vi "CRYUnflatten Data SC.vi"(10 "Unflatten data":string) -> (0 "Error?":bool, 2 "Data out":T3={"Name"="", "Curve"=[], "X data"=1, "Y data"=1, "Z data"=1, "X axis"=0, "Y axis"=1, "Z axis"=1, "X unit"="Hz", "Y unit"="", "Z unit"="deg.", "X dB ref"=1.0, "Y dB ref"=1.0, "Z dB ref"=1.0, "single val"=FALSE, "protected"=FALSE, "display X"=TRUE, "display Y"=TRUE, "display Z"=TRUE, "Plot Settings"={"Color"=0, "Interpolation"=2, "Point Style"=0, "Line Style"=0, "Point Color"=0, "Line Width"=0, "Bar Plot Style"=0, "Fill To"=-1}, "Test Info"=""} {"Z data" items=["dB", "Lin", "Pwr"]; "X data" items=["dB", "Lin", "Pwr"]; "Y data" items=["dB", "Lin", "Pwr"]; "Z dB ref" format="%.1f"; "Z axis" items=["Log", "Lin"]; "X dB ref" format="%.1f"; "X axis" items=["Log", "Lin"]; "Y axis" items=["Log", "Lin"]; "Y dB ref" format="%.1f"; "Curve"."z" format="%.2f"; "Curve"."y" format="%.2f"; "Curve"."x" format="%.2f"}, 3 "Header info out":T5={"Data type"="Data            ", "Version"=1, "Dimensions"=0, "Curve name"="Data            ", "Reserved"="Data            "})   [LabVIEW 2013]
uses:
  Typedef Control/CRYData Cluster SC.ctl
  Typedef Control/CRYAxis Unit Type.ctl
panel:
  in  "Datum 2.0":T1={"curve name"="", "Curve"=[], "Xdata"=0, "Ydata"=0, "Zdata"=0, "Xaxis"=0, "Yaxis"=0, "Zaxis"=0, "Xunit Prefix"="", "Yunit Prefix"="", "Zunit Prefix"="", "Xunit name"="", "Yunit name"="", "Zunit name"="", "X dB ref"=1.0, "Y dB ref"=1.0, "Z dB ref"=1.0, "single val"=FALSE} {"Z dB ref" format="%.1f"; "Y dB ref" format="%.1f"; "X dB ref" format="%.1f"; "Curve"."z" format="%.2f"; "Curve"."y" format="%.2f"; "Curve"."x" format="%.2f"}
  in  "Datum 3.0":T2={"curve name"="", "Curve"=[], "Xdata"=0, "Ydata"=0, "Zdata"=0, "Xaxis"=0, "Yaxis"=0, "Zaxis"=0, "Xunit Prefix"="", "Yunit Prefix"="", "Zunit Prefix"="", "Xunit name"="", "Yunit name"="", "Zunit name"="", "X dB ref"=1.0, "Y dB ref"=1.0, "Z dB ref"=1.0, "single val"=FALSE, "protected"=FALSE, "display X"=TRUE, "display Y"=TRUE, "display Z"=TRUE, "Plot Settings"={"Color"=0}} {"Z dB ref" format="%.1f"; "Y dB ref" format="%.1f"; "X dB ref" format="%.1f"; "Curve"."z" format="%.2f"; "Curve"."y" format="%.2f"; "Curve"."x" format="%.2f"}
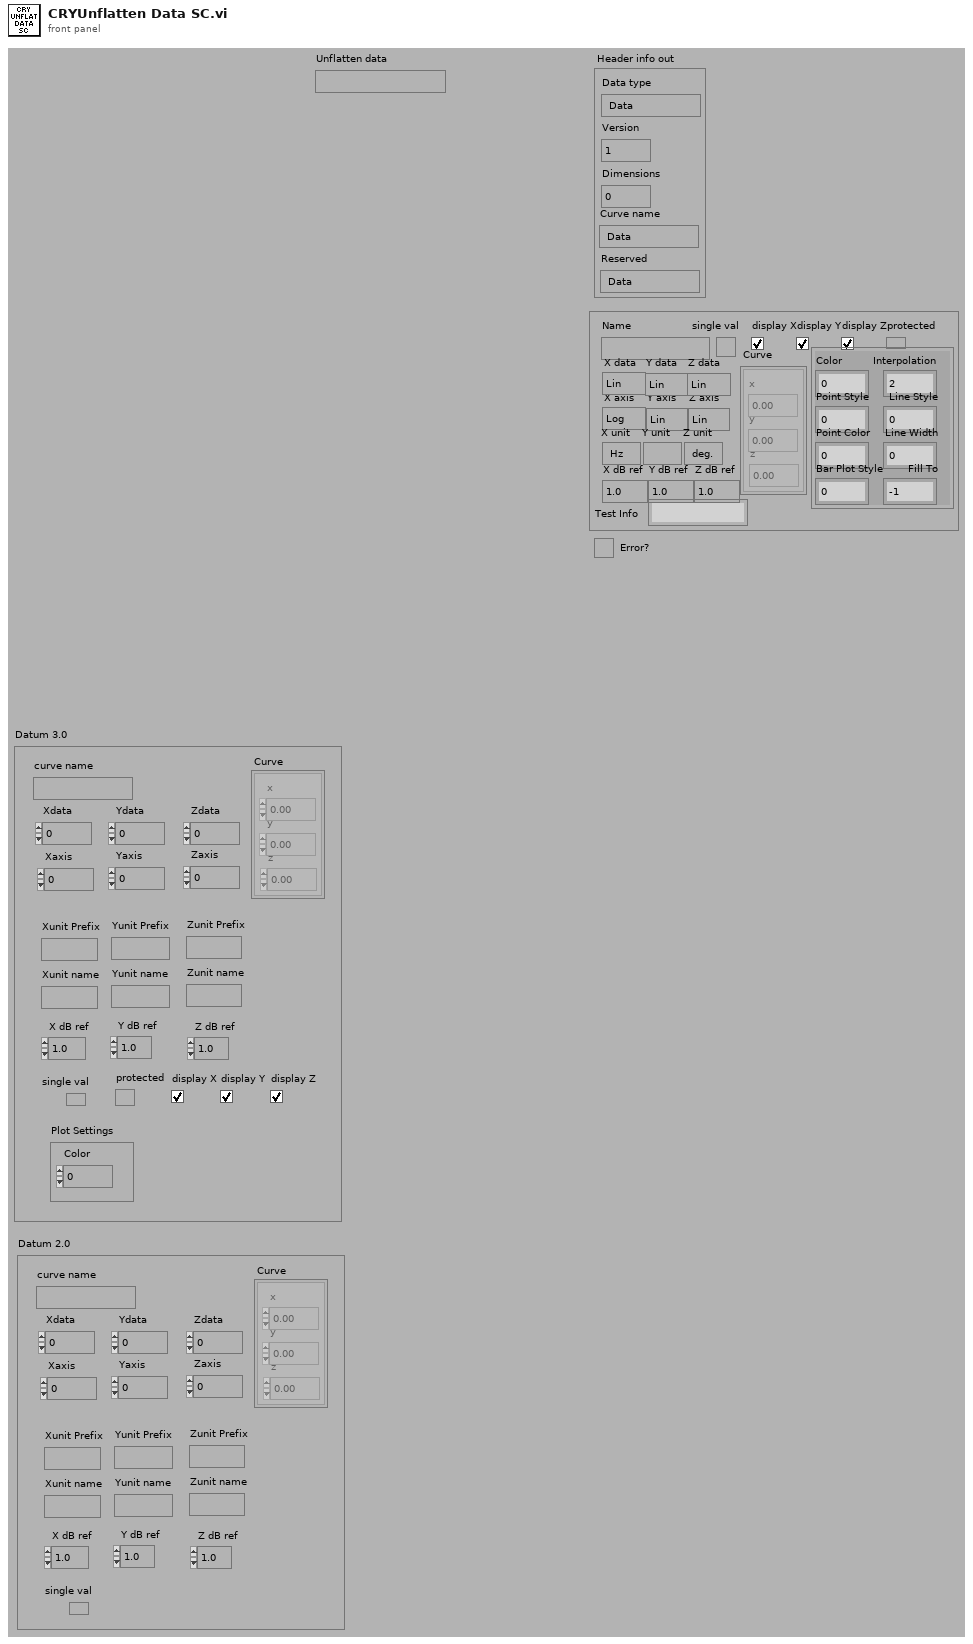
[diagram p1: front panel]
types:
  T1 = cluster{"curve name":string, "Curve":cluster{"x":dbl, "y":dbl, "z":dbl}[], "Xdata":u16, "Ydata":u16, "Zdata":u16, "Xaxis":u16, "Yaxis":u16, "Zaxis":u16, "Xunit Prefix":string, "Yunit Prefix":string, "Zunit Prefix":string, "Xunit name":string, "Yunit name":string, "Zunit name":string, "X dB ref":dbl, "Y dB ref":dbl, "Z dB ref":dbl, "single val":bool}
  T2 = cluster{"curve name":string, "Curve":cluster{"x":dbl, "y":dbl, "z":dbl}[], "Xdata":u16, "Ydata":u16, "Zdata":u16, "Xaxis":u16, "Yaxis":u16, "Zaxis":u16, "Xunit Prefix":string, "Yunit Prefix":string, "Zunit Prefix":string, "Xunit name":string, "Yunit name":string, "Zunit name":string, "X dB ref":dbl, "Y dB ref":dbl, "Z dB ref":dbl, "single val":bool, "protected":bool, "display X":bool, "display Y":bool, "display Z":bool, "Plot Settings":cluster{"Color":u32}}
  T3 = typedef "CRYData Cluster SC.ctl" = cluster{"Name":string, "Curve":cluster{"x":dbl, "y":dbl, "z":dbl}[], "X data":T4, "Y data":T4, "Z data":T4, "X axis":u16, "Y axis":u16, "Z axis":u16, "X unit":string, "Y unit":string, "Z unit":string, "X dB ref":dbl, "Y dB ref":dbl, "Z dB ref":dbl, "single val":bool, "protected":bool, "display X":bool, "display Y":bool, "display Z":bool, "Plot Settings":cluster{"Color":u32, "Interpolation":u8, "Point Style":u8, "Line Style":u8, "Point Color":u32, "Line Width":u8, "Bar Plot Style":u8, "Fill To":i16}, "Test Info":string}
  T4 = typedef "CRYAxis Unit Type.ctl" = u16
  T5 = cluster{"Data type":string, "Version":u16, "Dimensions":u8, "Curve name":string, "Reserved":string}
  T6 = cluster{"curve name":string, "Curve":cluster{"x":dbl, "y":dbl, "z":dbl}[], "Xdata":u16, "Ydata":u16, "Zdata":u16, "Xaxis":u16, "Yaxis":u16, "Zaxis":u16, "Xunit name":string, "Yunit name":string, "Zunit name":string, "X dB ref":dbl, "Y dB ref":dbl, "Z dB ref":dbl, "single val":bool, "protected":bool, "display X":bool, "display Y":bool, "display Z":bool, "Plot Settings":cluster{"Color":u32, "Interpolation":u8, "Point Style":u8, "Line Style":u8, "Point Color":u32, "Line Width":u8, "Bar Plot Style":u8, "Fill To":i16}, "Test Info":string}
  T7 = cluster{"Color":u32, "Interpolation":u8, "Point Style":u8, "Line Style":u8, "Point Color":u32, "Line Width":u8, "Bar Plot Style":u8, "Fill To":i16}
  T8 = cluster{"unsigned byte array[0]":u8, "unsigned byte array[1]":u8, "unsigned byte array[2]":u8}
  T9 = cluster{"substring":string, u16, "unsigned byte array[2]":u8, "Unflatten data":string, "Unflatten data":string}
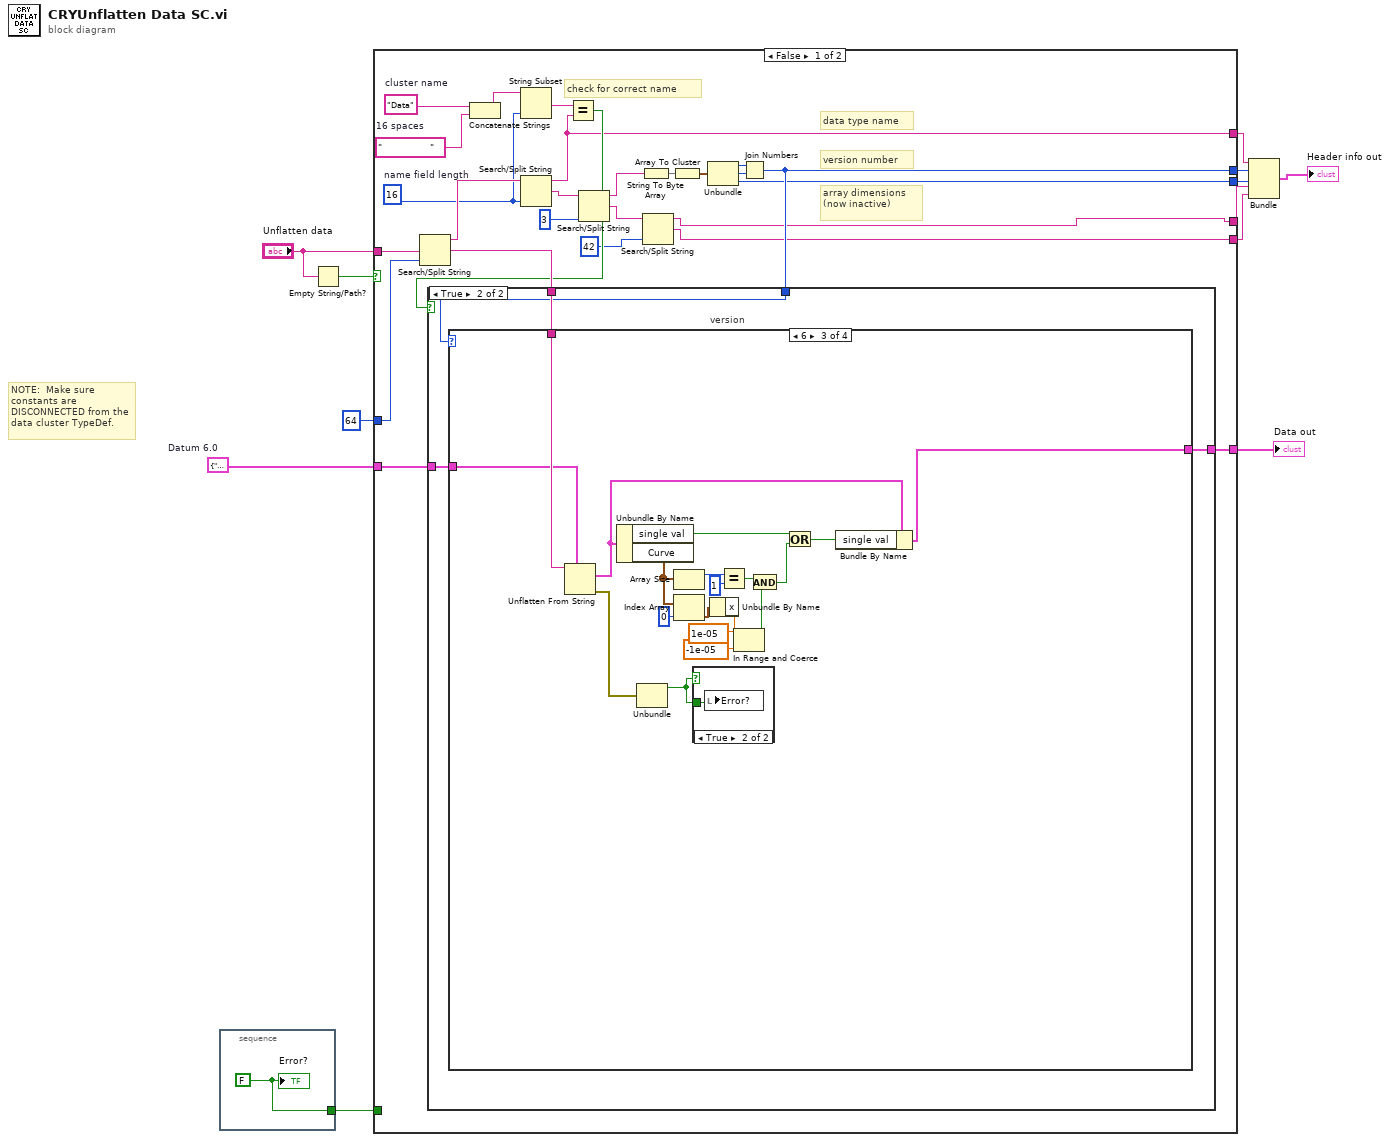
[diagram p0: block diagram]
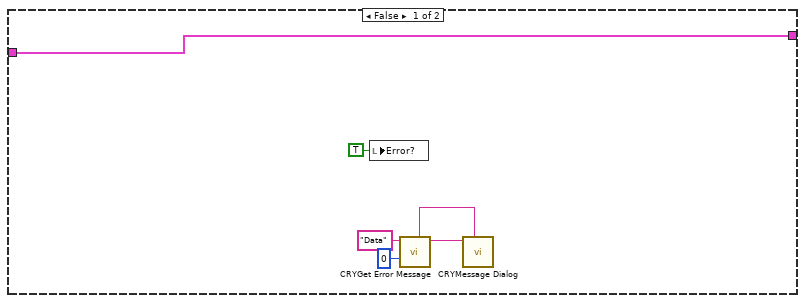
[diagram p2: hidden frame]
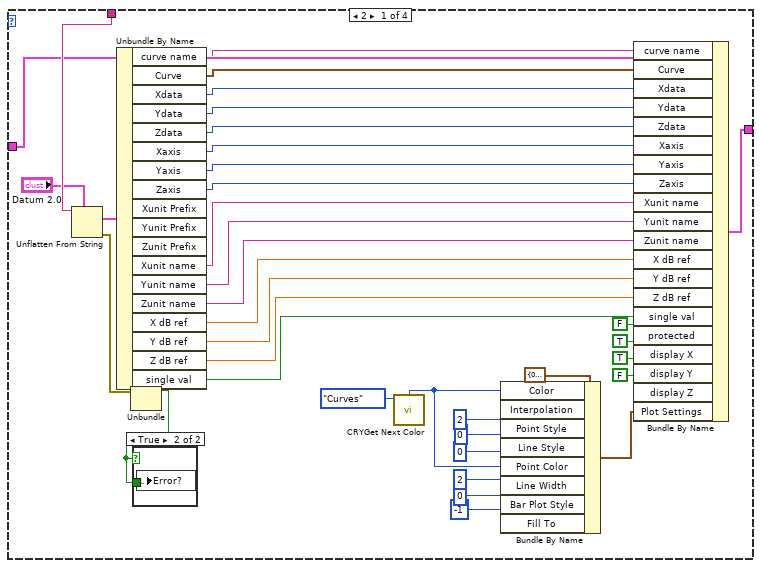
[diagram p3: hidden frame]
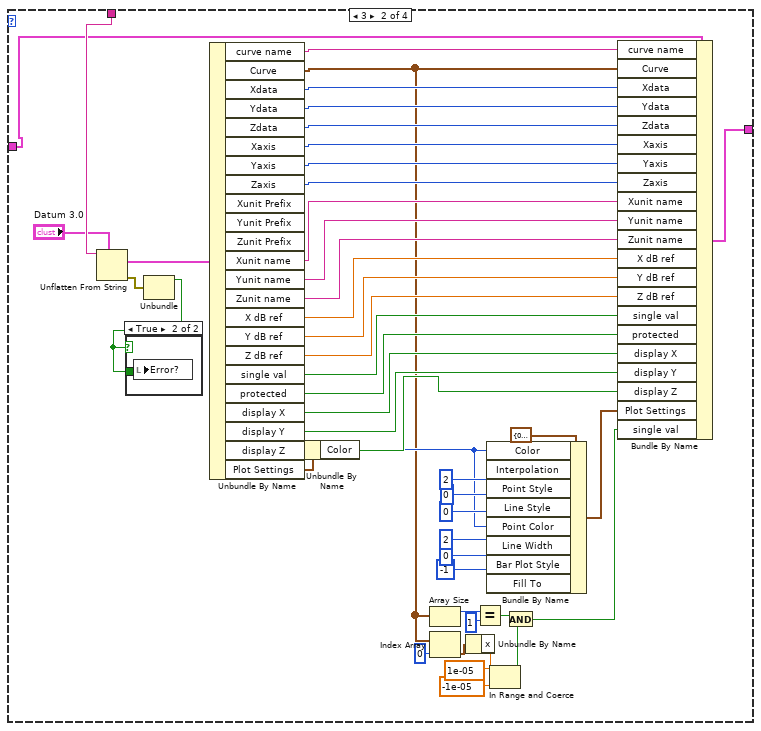
[diagram p5: hidden frame]
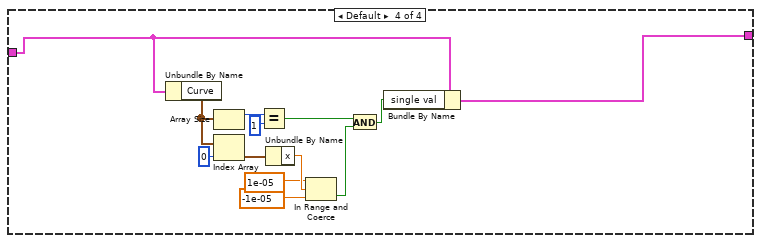
[diagram p8: hidden frame]
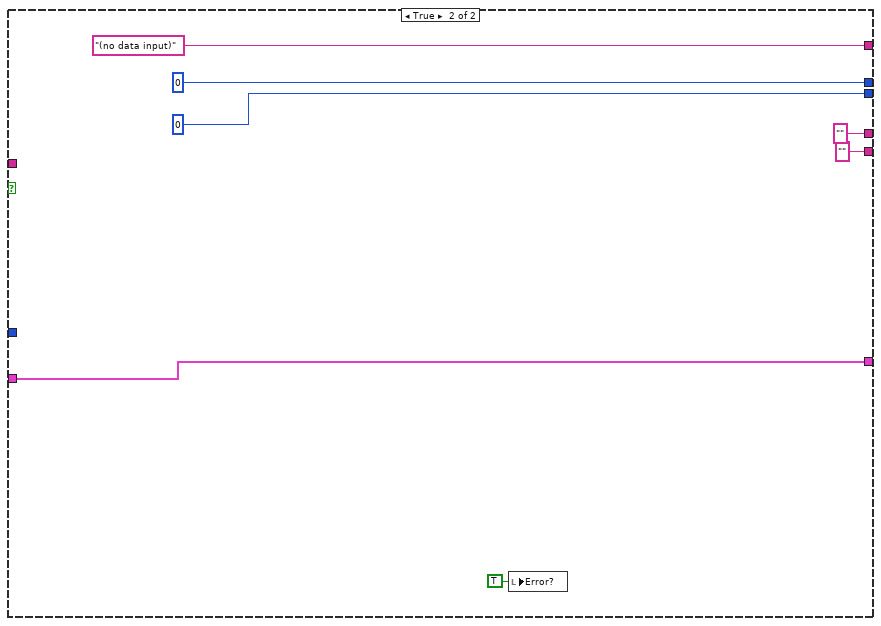
[diagram p9: hidden frame]
diagram:
  w2 = T6 {"curve name"="", "Curve"=[], "Xdata"=0, "Ydata"=0, "Zdata"=0, "Xaxis"=0, "Yaxis"=0, "Zaxis"=0, "Xunit name"="", "Yunit name"="", "Zunit name"="", "X dB ref"=0.0, "Y dB ref"=0.0, "Z dB ref"=0.0, "single val"=FALSE, "protected"=FALSE, "display X"=FALSE, "display Y"=FALSE, "display Z"=FALSE, "Plot Settings"={"Color"=0, "Interpolation"=0, "Point Style"=0, "Line Style"=0, "Point Color"=0, "Line Width"=0, "Bar Plot Style"=0, "Fill To"=0}, "Test Info"=""}  # Datum 6.0
  # "NOTE:  Make sure constants are DISCONNECTED from the data cluster TypeDef."
  n1 = stacked-sequence {
    tunnel: [w13] -> w1
    frame #0 {
      w13 = FALSE
      "Error?" <- w13
    }
  }
  n2 = Empty String/Path?(string/path="Unflatten data") -> (empty?=w11:bool)
  n3 = case shown="False" w11 {
    tunnel: "Unflatten data" -> [w39 _]
    tunnel: 64 ("header length") -> [w33 _]
    tunnel: [w30 u16 0] -> w8
    tunnel: [w23 u8 0] -> w9
    tunnel: [w24 "(no data input)" ("substring")] -> w7
    tunnel: [w22 w170] -> w3
    tunnel: w2 -> [w21 w170]
    tunnel: [w15 "" ("Unflatten data")] -> w5
    tunnel: [w14 "" ("Unflatten data")] -> w4
    tunnel: w1 -> [_ _]
    frame False {
      w28 = "                "  # 16 spaces
      w29 = "Data"  # cluster name
      w26 = 16  # name field length
      # "check for correct name"
      # "array dimensions\n(now inactive)"
      # "version number"
      # "data type name"
      n4 = Search/Split String(string=w39, offset (0)=w33) -> (substring before match=w32:string, match + rest of string=w34:string)  [unwired: 2 out]
      n5 = Concatenate Strings(w29, w28) -> (w27:string)
      n6 = String Subset(string=w27, length (rest)=w26) -> (substring=w25:string)  [unwired: 1 out]
      n7 = Search/Split String(string=w32, offset (0)=w26) -> (substring before match=w24:string, match + rest of string=w20:string)  [unwired: 2 out]
      n8 = Equal?(x=w25, y=w24) -> (x = y?=w31:bool)
      n9 = Search/Split String(string=w20, offset (0)=3 ("name field length")) -> (substring before match=w18:string, match + rest of string=w17:string)  [unwired: 2 out]
      n10 = String To Byte Array(string=w18) -> (unsigned byte array=w38:u8[])
      n11 = Search/Split String(string=w17, offset (0)=42 ("name field length")) -> (substring before match=w15:string, match + rest of string=w14:string)  [unwired: 2 out]
      n12 = Array To Cluster(array=w38) -> (cluster=w37:T8)
      n13 = Unbundle(w37) -> ("unsigned byte array[0]"=w36:u8, "unsigned byte array[1]"=w35:u8, "unsigned byte array[2]"=w23:u8)
      n14 = Join Numbers(hi=w36, lo=w35) -> ((hi.lo)=w30:u16)
      n15 = case shown="True" w31 {
        tunnel: w34 -> [_ w49]
        tunnel: w30 -> [_ w48]
        tunnel: [w45 w47] -> w22
        tunnel: w21 -> [w45 w46]
        frame False {
          n16 = local write "Error?"(TRUE ("Error?")) -> ()
          n17 = call "CRYGet Error Message.vi"("Error No"=0, "Kind"="Data") -> ("Message"=w43:string, "Window Title"=w44:string)  [unwired: 4 in, 4 out]
          n18 = call "CRYMessage Dialog.vi"("Window Title"=w44, "Message Content"=w43) -> ()  [unwired: 8 in, 2 out]
        }
        frame True {
          n19 = case "version" shown="6" w48 {
            tunnel: w49 -> [w85 w132 w137 _]
            tunnel: [w68 w110 w136 w154] -> w47
            tunnel: w46 -> [w83 w129 w135 w155]
            frame 2 {
              n20 = Unflatten From String(type="Datum 2.0", binary string=w85) -> (value=w84:T1, error out=w50:errorcluster)  [unwired: 1 in, 3 out]
              n21 = Unbundle By Name(w84) -> ("curve name"=w82:string, "Curve"=w81:cluster{"x":dbl, "y":dbl, "z":dbl}[], "Xdata"=w80:u16, "Ydata"=w79:u16, "Zdata"=w78:u16, "Xaxis"=w77:u16, "Yaxis"=w76:u16, "Zaxis"=w75:u16, "Xunit name"=w74:string, "Yunit name"=w73:string, "Zunit name"=w72:string, "X dB ref"=w71:dbl, "Y dB ref"=w70:dbl, "Z dB ref"=w62:dbl, "single val"=w69:bool)  [unwired: 3 out]
              n22 = Unbundle(w50) -> ("status"=w51:bool)  [unwired: 2 out]
              n23 = case shown="True" w51 {
                tunnel: w51 -> [_ w86]
                frame False {
                }
                frame True {
                  n24 = local write "Error?"(w86) -> ()
                }
              }
              n25 = call "CRYGet Next Color.vi"("Type"=enum16{"Curves", "Values", "Results", "WFM"}."Curves") -> ("Color"=w53:u32)  [unwired: 10 out]
              n26 = Bundle By Name(cluster=T7 {"Color"=0, "Interpolation"=0, "Point Style"=0, "Line Style"=0, "Point Color"=0, "Line Width"=0, "Bar Plot Style"=0, "Fill To"=0} ("Plot Settings"), "Color"=w53, "Interpolation"=u8 2 ("Plot Settings.Interpolation"), "Point Style"=u8 0 ("Plot Settings.Point Style"), "Line Style"=u8 0 ("Plot Settings.Line Style"), "Point Color"=w53, "Line Width"=u8 2 ("Plot Settings.Line Width"), "Bar Plot Style"=u8 0 ("Plot Settings.Bar Plot Style"), "Fill To"=i16 -1 ("Plot Settings.Fill To")) -> (w54:T7)
              n27 = Bundle By Name(cluster=w83, "curve name"=w82, "Curve"=w81, "Xdata"=w80, "Ydata"=w79, "Zdata"=w78, "Xaxis"=w77, "Yaxis"=w76, "Zaxis"=w75, "Xunit name"=w74, "Yunit name"=w73, "Zunit name"=w72, "X dB ref"=w71, "Y dB ref"=w70, "Z dB ref"=w62, "single val"=w69, "protected"=FALSE, "display X"=TRUE, "display Y"=TRUE, "display Z"=FALSE, "Plot Settings"=w54) -> (w68:T6)
            }
            frame 3 {
              n28 = Unflatten From String(type="Datum 3.0", binary string=w132) -> (value=w130:T2, error out=w87:errorcluster)  [unwired: 1 in, 3 out]
              n29 = Unbundle(w87) -> ("status"=w88:bool)  [unwired: 2 out]
              n30 = case shown="True" w88 {
                tunnel: w88 -> [_ w133]
                frame False {
                }
                frame True {
                  n31 = local write "Error?"(w133) -> ()
                }
              }
              n32 = Unbundle By Name(w130) -> ("curve name"=w128:string, "Curve"=w90:cluster{"x":dbl, "y":dbl, "z":dbl}[], "Xdata"=w127:u16, "Ydata"=w126:u16, "Zdata"=w125:u16, "Xaxis"=w124:u16, "Yaxis"=w123:u16, "Zaxis"=w122:u16, "Xunit name"=w121:string, "Yunit name"=w120:string, "Zunit name"=w119:string, "X dB ref"=w118:dbl, "Y dB ref"=w117:dbl, "Z dB ref"=w109:dbl, "single val"=w116:bool, "protected"=w115:bool, "display X"=w114:bool, "display Y"=w113:bool, "display Z"=w112:bool, "Plot Settings"=w111:cluster{"Color":u32})  [unwired: 3 out]
              n33 = Unbundle By Name(w111) -> ("Color"=w102:u32)
              n34 = Array Size(array=w90) -> (size(s)=w94:i32)
              n35 = Index Array(array=w90, index=0 ("Index")) -> (element=w97:cluster{"x":dbl, "y":dbl, "z":dbl})
              n36 = Unbundle By Name(w97) -> ("x"=w98:dbl)
              n37 = Equal?(x=w94, y=1) -> (x = y?=w96:bool)
              n38 = Bundle By Name(cluster=T7 {"Color"=0, "Interpolation"=0, "Point Style"=0, "Line Style"=0, "Point Color"=0, "Line Width"=0, "Bar Plot Style"=0, "Fill To"=0} ("Plot Settings"), "Color"=w102, "Interpolation"=u8 2 ("Plot Settings.Interpolation"), "Point Style"=u8 0 ("Plot Settings.Point Style"), "Line Style"=u8 0 ("Plot Settings.Line Style"), "Point Color"=w102, "Line Width"=u8 2 ("Plot Settings.Line Width"), "Bar Plot Style"=u8 0 ("Plot Settings.Bar Plot Style"), "Fill To"=i16 -1 ("Plot Settings.Fill To")) -> (w100:T7)
              n39 = In Range and Coerce(upper limit=1e-05, x=w98, lower limit=-1e-05) -> (In Range?=w99:bool)  [unwired: 1 out]
              n40 = And(x=w96, y=w99) -> (x .and. y?=w89:bool)
              n41 = Bundle By Name(cluster=w129, "curve name"=w128, "Curve"=w90, "Xdata"=w127, "Ydata"=w126, "Zdata"=w125, "Xaxis"=w124, "Yaxis"=w123, "Zaxis"=w122, "Xunit name"=w121, "Yunit name"=w120, "Zunit name"=w119, "X dB ref"=w118, "Y dB ref"=w117, "Z dB ref"=w109, "single val"=w116, "protected"=w115, "display X"=w114, "display Y"=w113, "display Z"=w112, "Plot Settings"=w100, "single val"=w89) -> (w110:T6)
            }
            frame 6 {
              n42 = Unflatten From String(type=w135, binary string=w137) -> (value=w134:T6, error out=w139:errorcluster)  [unwired: 1 in, 3 out]
              n43 = Unbundle By Name(w134) -> ("single val"=w150:bool, "Curve"=w149:cluster{"x":dbl, "y":dbl, "z":dbl}[])
              n44 = Unbundle(w139) -> ("status"=w138:bool)  [unwired: 2 out]
              n45 = Array Size(array=w149) -> (size(s)=w143:i32)
              n46 = Index Array(array=w149, index=0 ("Index")) -> (element=w146:cluster{"x":dbl, "y":dbl, "z":dbl})
              n47 = case shown="True" w138 {
                tunnel: w138 -> [_ w153]
                frame False {
                }
                frame True {
                  n48 = local write "Error?"(w153) -> ()
                }
              }
              n49 = Unbundle By Name(w146) -> ("x"=w147:dbl)
              n50 = Equal?(x=w143, y=1) -> (x = y?=w145:bool)
              n51 = In Range and Coerce(upper limit=1e-05, x=w147, lower limit=-1e-05) -> (In Range?=w148:bool)  [unwired: 1 out]
              n52 = And(x=w145, y=w148) -> (x .and. y?=w151:bool)
              n53 = Or(x=w150, y=w151) -> (x .or. y?=w152:bool)
              n54 = Bundle By Name(cluster=w134, "single val"=w152) -> (w136:T6)
            }
            frame Default {
              n55 = Unbundle By Name(w155) -> ("Curve"=w165:cluster{"x":dbl, "y":dbl, "z":dbl}[])
              n56 = Array Size(array=w165) -> (size(s)=w159:i32)
              n57 = Index Array(array=w165, index=0 ("Index")) -> (element=w162:cluster{"x":dbl, "y":dbl, "z":dbl})
              n58 = Equal?(x=w159, y=1) -> (x = y?=w161:bool)
              n59 = Unbundle By Name(w162) -> ("x"=w163:dbl)
              n60 = In Range and Coerce(upper limit=1e-05, x=w163, lower limit=-1e-05) -> (In Range?=w164:bool)  [unwired: 1 out]
              n61 = And(x=w161, y=w164) -> (x .and. y?=w166:bool)
              n62 = Bundle By Name(cluster=w155, "single val"=w166) -> (w154:T6)
            }
          }
        }
      }
    }
    frame True {
      n63 = local write "Error?"(TRUE ("Error?")) -> ()
    }
  }
  "Data out" <- w3
  n64 = Bundle("substring"=w7, w8, "unsigned byte array[2]"=w9, "Unflatten data"=w5, "Unflatten data"=w4) -> (→"Header info out":T9)  [unwired: 1 out]
